vi "SectionA04_Week8_Stus.vi"() -> ()   [LabVIEW 2013]
panel:
  out "Samples In Queue":u8(slide) scale=0.0..100.0
  out "Loop Rate":u32
  in  "Loop Speed":u16(ring) items=["Same as Producer"=50, "Max Speed"=0, "2x as Producer"=25, "1/2 as Producer"=100, "1/20 as Producer"=1000]
  out "Queue Loop":dbl(graph)
  in  "Amplitude":dbl
  out "Producer Loop":dbl(graph)
  in  "Switch":bool
  out "# of Samples":i32
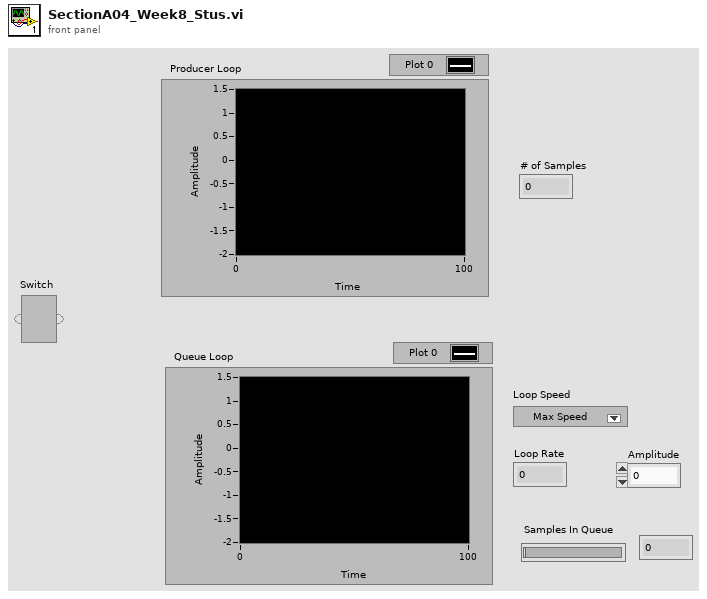
[diagram p1: front panel]
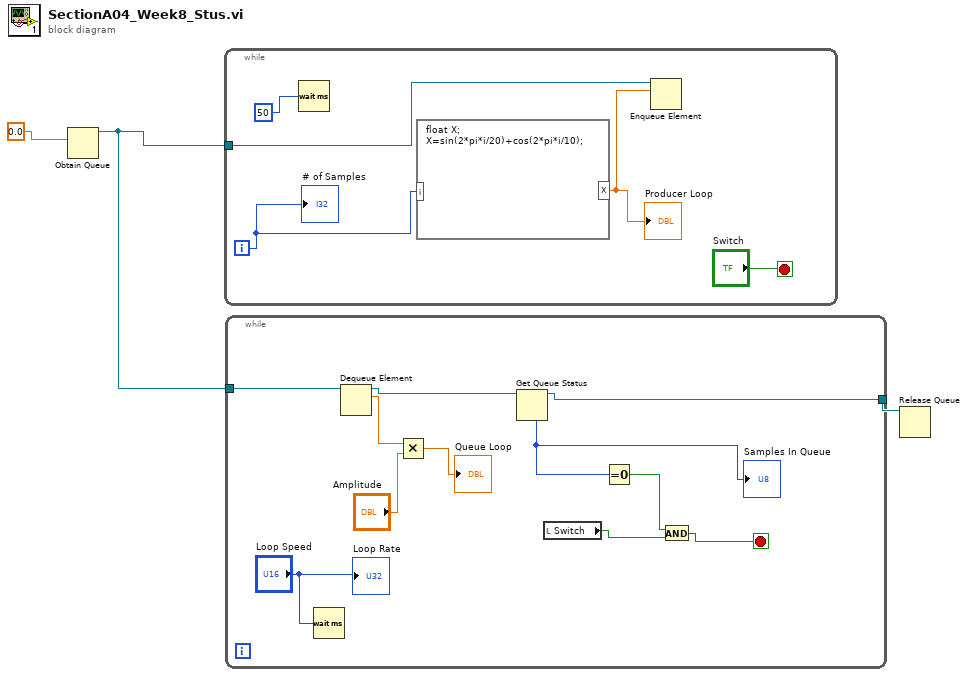
[diagram p0: block diagram]
diagram:
  n1 = Obtain Queue(element data type=0.0) -> (queue out=w3:refnum<queue>)  [unwired: 4 in, 2 out]
  n2 = while {
    tunnel: w3 -> [w8]
    i -> [w7]
    stop <- "Switch" stop-if-true
    n3 = Wait (ms)(milliseconds to wait=50) -> ()  [unwired: 1 out]
    n4 = formula code="float X;\nX=sin(2*pi*i/20)+cos(2*pi*i/10);"("i"=w7) -> ("X"=w6:dbl)
    "Producer Loop" <- w6
    n5 = Enqueue Element(queue=w8, element=w6) -> ()  [unwired: 2 in, 3 out]
    "# of Samples" <- w7
  }
  n6 = while {
    tunnel: w3 -> [w19]
    tunnel: [w17] -> w2
    stop <- w12 stop-if-true
    n7 = Wait (ms)(milliseconds to wait="Loop Speed") -> ()  [unwired: 1 out]
    n8 = Dequeue Element(queue=w19) -> (queue out=w18:refnum<queue>, element=w16:dbl)  [unwired: 2 in, 2 out]
    n9 = Multiply(x=w16, y="Amplitude") -> (x*y=→"Queue Loop":dbl)
    n10 = Get Queue Status(queue=w18) -> (queue out=w17:refnum<queue>, # elements in queue=w9:i32)  [unwired: 2 in, 6 out]
    "Samples In Queue" <- w9
    n11 = local read "Switch"() -> (w10:bool)
    n12 = Equal To 0?(x=w9) -> (x = 0?=w11:bool)
    n13 = And(x=w11, y=w10) -> (x .and. y?=w12:bool)
    "Loop Rate" <- "Loop Speed"
  }
  n14 = Release Queue(queue=w2) -> ()  [unwired: 2 in, 3 out]
